vi "Extract results.vi"(8 "error in (no error)":errorcluster, 9 "Results temp folder":path, 10 "APG Config":T1) -> (0 "error out":errorcluster)   [LabVIEW 2013, in "Manipulate IPF.lvlib"]
uses:
  Manipulate IPF.lvlib
  Settings/type_def/APG Config.ctl
  Pack Data/type_def/file types.ctl
  type_def/IPF cmd.ctl
  Pack Data/Pack Files.lvlib
  Settings/APG_settings.lvlib
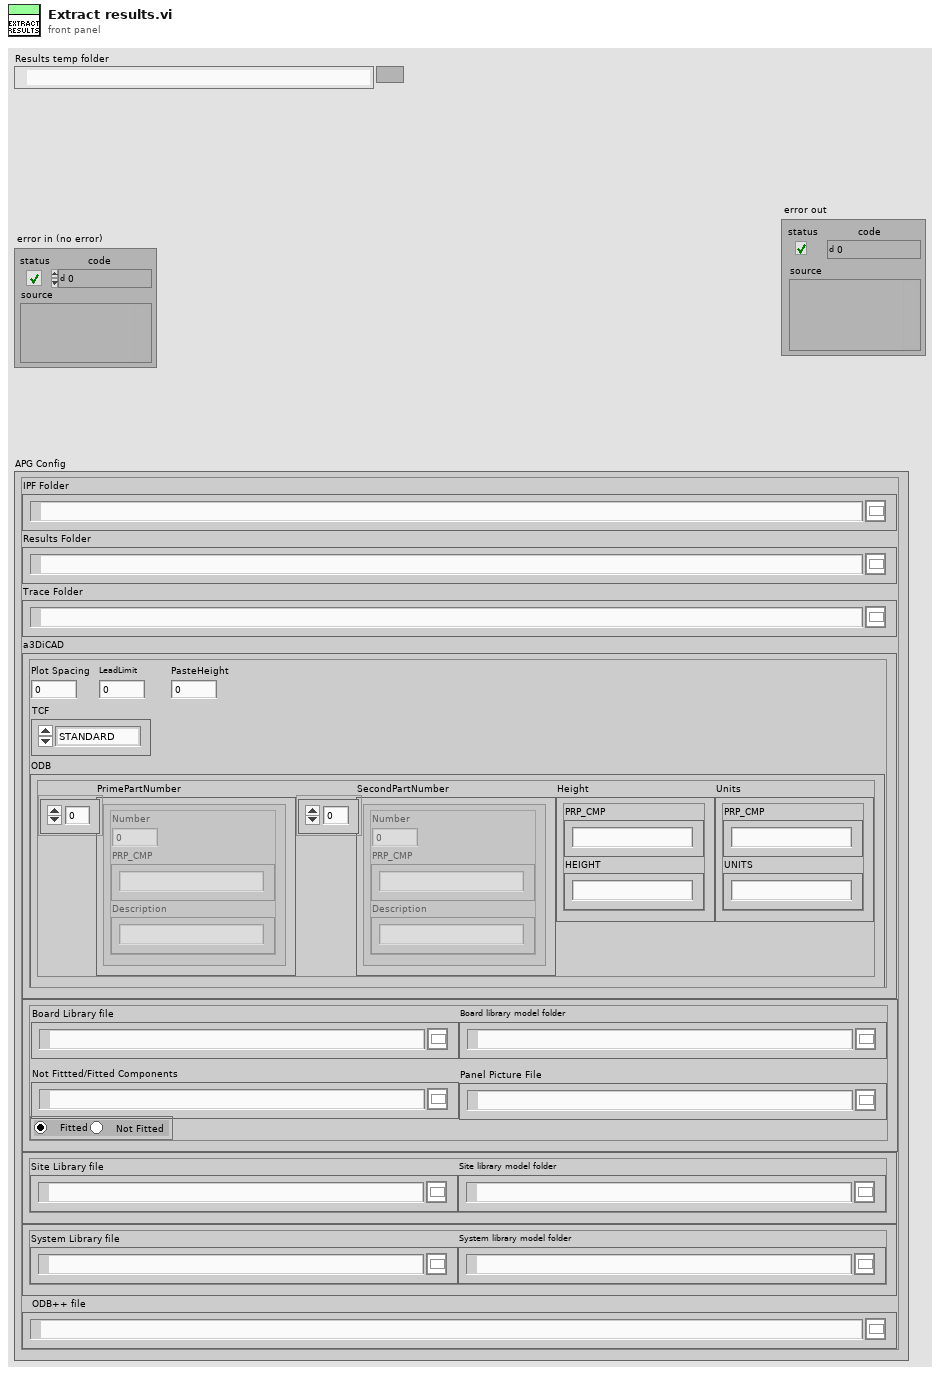
[diagram p1: front panel]
types:
  T1 = typedef "APG_settings.lvlib/APG Config.ctl" = cluster{"IPF Folder":path, "Results Folder":path, "Trace Folder":path, "a3DiCAD":cluster{"Plot Spacing":dbl, "TCF":enum16{"STANDARD", "PASTE", "LEAD"}, "LeadLimit":u32, "a3DiCADDebug":bool, "ODB":cluster{"PrimePartNumber":cluster{"Number":u32, "PRP_CMP":string, "Description":string}[], "SecondPartNumber":cluster{"Number":u32, "PRP_CMP":string, "Description":string}[], "Height":cluster{"PRP_CMP":string, "HEIGHT":string}, "Units":cluster{"PRP_CMP":string, "UNITS":string}}, "PasteHeight":dbl}, "a3DiCADcfg":path, "Board Library":cluster{"Board Library file":path, "Board library model folder":path, "Not Fittted/Fitted Components":path, "Panel Picture File":path, "Components":enum32{"Fitted", "Not Fitted "}}, "Site Library":cluster{"Site Library file":path, "Site library model folder":path}, "System Library":cluster{"System Library file":path, "System library model folder":path}, "ODB++ file":path}
  T2 = typedef "Manipulate IPF.lvlib/IPF cmd.ctl" = enum16{"New IPF", "Edit IPF", "Copy IPF", "Rename IPF", "Delete IPF", "Reload IPF", "Load all IPF"}
  T3 = typedef "Pack Files.lvlib/file types.ctl" = enum16{"ODB", "TCF", "CAD Outline", "Config", "Inspection Prog", "a3Di-bin", "Results", "CAD Labels", "CAD Pads", "calScan_fid", "calScan_cal-tab", "PCB_SerialNumber", "CAD_Assembly", "Version", "Old Results", "CAD Picture", "Old TCF"}
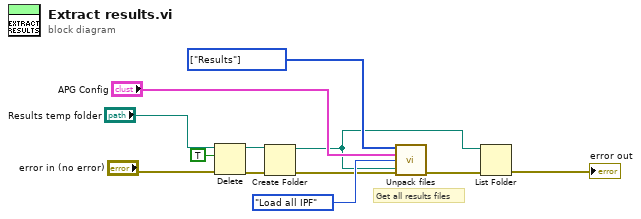
[diagram p0: block diagram]
diagram:
  w11 = T3[] [enum."Results"] items=["ODB", "TCF", "CAD Outline", "Config", "Inspection Prog", "a3Di-bin", "Results", "CAD Labels", "CAD Pads", "calScan_fid", "calScan_cal-tab", "PCB_SerialNumber", "CAD_Assembly", "Version", "Old Results", "CAD Picture", "Old TCF"] ("IPF files[]")
  # "Get all results files"
  n1 = Delete(path (use dialog)="Results temp folder", entire hierarchy (F)=TRUE, error in="error in (no error)") -> (deleted path=w3:path, error out=w5:errorcluster)  [unwired: 2 in, 1 out]
  n2 = Create Folder(path (use dialog)=w3, error in=w5) -> (created path=w1:path, error out=w4:errorcluster)  [unwired: 1 in, 1 out]
  n3 = call "Unpack files.vi"("IPF files[]"=w11, "APG Config"="APG Config", "IPF cmd"=IPF_cmd."Load all IPF", "Destination folder"=w1, "error in (no error)"=w4) -> ("error out"=w10:errorcluster)  [unwired: 10 in]
  n4 = List Folder(path=w1, error in=w10) -> (error out=→"error out":errorcluster)  [unwired: 2 in, 3 out]
